vi "Format Button Message.vi"(7 "Switch":T1=enum."SW201 - My Cycle") -> (8 "Switch Message":string)   [LabVIEW 2014]
uses:
  type defs/HEUI Switches.ctl
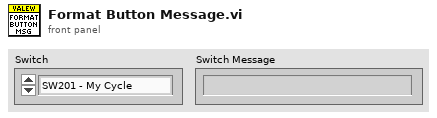
[diagram p1: front panel]
types:
  T1 = typedef "HEUI Switches.ctl" = enum16{"Switch Off", "SW201 - My Cycle", "SW202 - Delay Wash", "SW203 - Extra Rinse", "SW204 - Signal Adjust", "SW205 - Spin", "SW206 - Deep Rinse", "SW207 - Soil", "SW208 - Auto Soak", "SW209 - Temp", "SW210 - Warm Rinse", "SW211 - Deep Fill", "SW212 - Stains", "SW213 - Power", "SW214 - Start/Pause", "SW215", "SW216"}
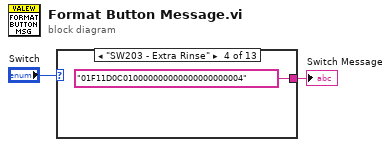
[diagram p0: block diagram]
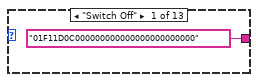
[diagram p2: hidden frame]
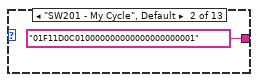
[diagram p3: hidden frame]
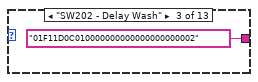
[diagram p4: hidden frame]
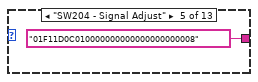
[diagram p5: hidden frame]
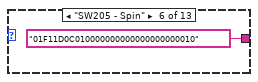
[diagram p6: hidden frame]
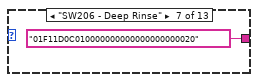
[diagram p7: hidden frame]
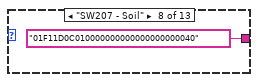
[diagram p8: hidden frame]
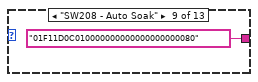
[diagram p9: hidden frame]
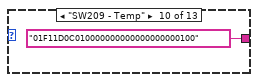
[diagram p10: hidden frame]
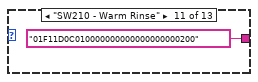
[diagram p11: hidden frame]
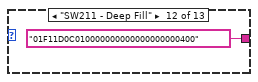
[diagram p12: hidden frame]
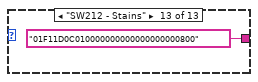
[diagram p13: hidden frame]
diagram:
  n1 = case shown="\"SW203 - Extra Rinse\"" "Switch" {
    tunnel: ["01F11D0C000000000000000000000000" ("Message") "01F11D0C010000000000000000000001" ("Message") "01F11D0C010000000000000000000002" ("Message") "01F11D0C010000000000000000000004" ("Message") "01F11D0C010000000000000000000008" ("Message") "01F11D0C010000000000000000000010" ("Message") "01F11D0C010000000000000000000020" ("Message") "01F11D0C010000000000000000000040" ("Message") "01F11D0C010000000000000000000080" ("Message") "01F11D0C010000000000000000000100" ("Message") "01F11D0C010000000000000000000200" ("Message") "01F11D0C010000000000000000000400" ("Message") "01F11D0C010000000000000000000800" ("Message")] -> w1
    frame "Switch Off" {
    }
    frame "SW201 - My Cycle", Default {
    }
    frame "SW202 - Delay Wash" {
    }
    frame "SW203 - Extra Rinse" {
    }
    frame "SW204 - Signal Adjust" {
    }
    frame "SW205 - Spin" {
    }
    frame "SW206 - Deep Rinse" {
    }
    frame "SW207 - Soil" {
    }
    frame "SW208 - Auto Soak" {
    }
    frame "SW209 - Temp" {
    }
    frame "SW210 - Warm Rinse" {
    }
    frame "SW211 - Deep Fill" {
    }
    frame "SW212 - Stains" {
    }
  }
  "Switch Message" <- w1
